vi "citTemplate.Loop Example.vi"() -> ()   [LabVIEW 2015]
uses:
  citTemplate.errData.ctl
  EventLog/EventLog.EventSource.ctl
panel:
  out "_loop":i32(ring)=4
types:
  T1 = typedef "citTemplate.errData.ctl" = cluster{"ts":timestamp, "src":T2, "instance":i32, "action":string, "error":errorcluster, "unconfirmed":bool}
  T2 = typedef "EventLog.EventSource.ctl" = enum16{"All", "Gui", "DB1", "DB2", "DB3", "PLC1", "PLC2", "PLC3"}
  T3 = enum32{"idle", "constructor", "destructor", "--- Loop Name ---"}
  T4 = typedef "citTemplate.notifierHandle.ctl" = refnum<notifier>
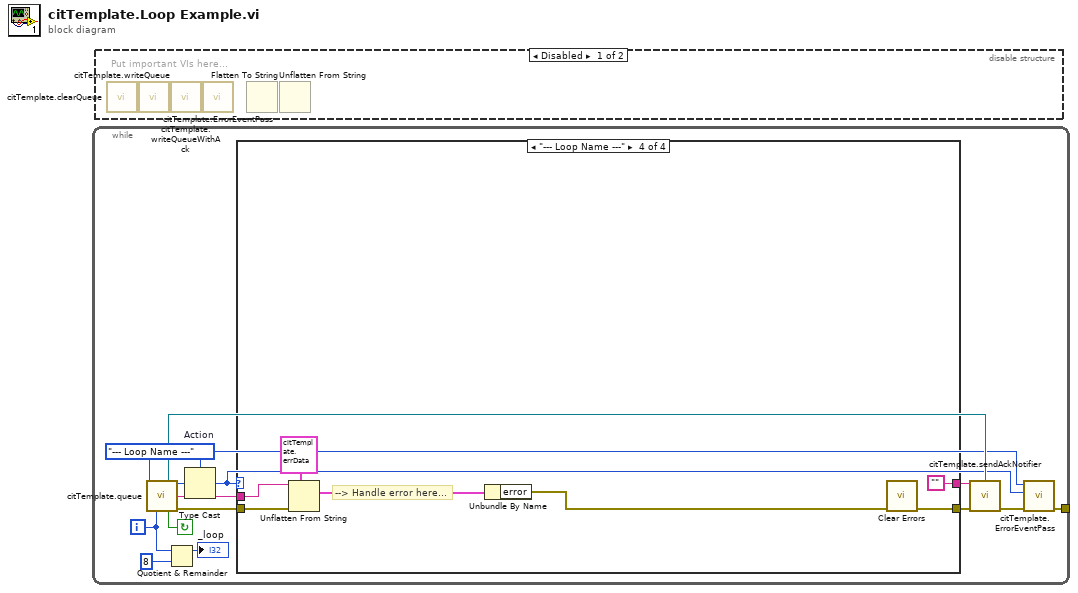
[diagram p0: block diagram]
diagram:
  n1 = while {
    tunnel: [w1] -> _
    i -> [w3]
    stop <- w10 continue-if-true
    w7 = T3."--- Loop Name ---"  # Action
    n2 = call "citTemplate.queue.vi"("event enum"=w7, "iteration (-1)"=w3) -> ("notifierHandle out"=w9:T4, "event out"=w13:u32, "(flatten) data out"=w12:string, "continue"=w10:bool, "error out"=w11:errorcluster)  [unwired: 3 in, 6 out]
    n3 = Quotient & Remainder(x=w3, y=8) -> (x-y*floor(x/y)=→"_loop":i32)  [unwired: 1 out]
    n4 = Type Cast(type=w7, x=w13) -> (*(type *) &x=w2:T3)
    n5 = case shown="\"--- Loop Name ---\"" w2 {
      tunnel: w12 -> [_ _ _ w22]
      tunnel: w11 -> [w14 w15 w16 w20]
      tunnel: [_ _ _ ""] -> w8
      tunnel: [w14 w15 w16 w21] -> w6
      frame "idle" {
      }
      frame "constructor" {
      }
      frame "destructor" {
      }
      frame "--- Loop Name ---" {
        # "--> Handle error here..."
        n6 = Unflatten From String(type=T1 {"ts"=timestamp(0 s since 1904-01-01), "src"=enum."All", "instance"=0, "action"="", "error"={"status"=FALSE, "code"=0, "source"=""}, "unconfirmed"=FALSE} ("ErrData"), binary string=w22, error in (no error)=w20) -> (value=w18:T1)  [unwired: 4 out]
        n7 = Unbundle By Name(w18) -> ("error"=w17:errorcluster)
        n8 = call <vilib>:"Clear Errors.vi"("error in (no error)"=w17) -> ("error out"=w21:errorcluster)  [unwired: 5 in, 1 out]
      }
    }
    n9 = call "citTemplate.sendAckNotifier.vi"("notification data"=w8, "notifierHandle in"=w9, "error in"=w6) -> ()  [unwired: 13 out]
    n10 = call "citTemplate.ErrorEventPass.vi"("error in"=w6, "action of error"=w2, "event in"=w7) -> ("error out"=w1:errorcluster)  [unwired: 2 in, 6 out]
  }
  n11 = disable-structure shown="Disabled" {
    frame Disabled {
      # "Put important VIs here..."
      n12 = call "citTemplate.clearQueue.vi"() -> ()  [unwired: 14 in, 2 out]
      n13 = call "citTemplate.writeQueue.vi"() -> ()  [unwired: 15 in, 1 out]
      n14 = call "citTemplate.writeQueueWithAck.vi"() -> ()  [unwired: 13 in, 3 out]
      n15 = call "citTemplate.ErrorEventPass.vi"() -> ()  [unwired: 11 in, 1 out]
      n16 = Flatten To String() -> ()  [unwired: 4 in, 3 out]
      n17 = Unflatten From String() -> ()  [unwired: 5 in, 3 out]
    }
    frame Enabled {
    }
  }
